vi "MFCConfigurationGlobal.vi"(6 "Index":i32, 7 "Action":T5=enum."Get", 11 "Set Value":T1) -> (3 "Value Out":T1)   [LabVIEW 2012]
uses:
  MFCConfigurationGlobalAction.ctl
  MFCConfiguration.ctl
  libs/Sierra-M100/Public/Controls/ValveState.ctl
  libs/Sierra-M100/Public/Controls/Gas.ctl
  libs/Sierra-M100/Public/Controls/Units.ctl
  libs/Sierra-M100/Sierra-M100.lvlib
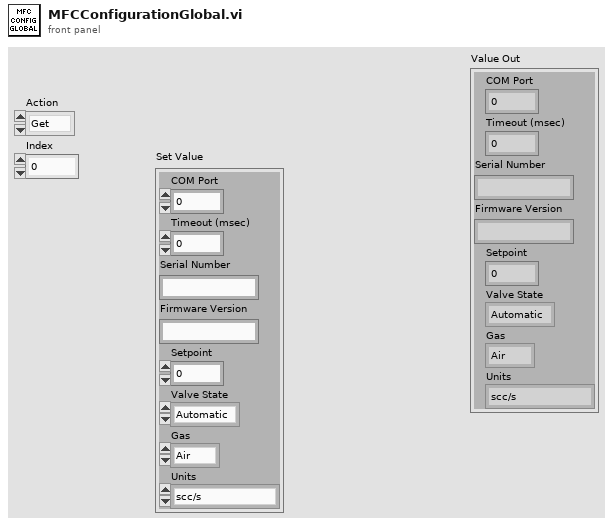
[diagram p1: front panel]
types:
  T1 = typedef "MFCConfiguration.ctl" = cluster{"COM Port":u32, "Timeout (msec)":u32, "Setpoint":dbl, "Valve State":T2, "Gas":T3, "Units":T4, "Serial Number":string, "Firmware Version":string}
  T2 = typedef "Sierra-M100.lvlib/ValveState.ctl" = enum16{"Automatic", "Closed", "Purge"}
  T3 = typedef "Sierra-M100.lvlib/Gas.ctl" = enum16{"Air", "Argon", "CO2", "CO", "Helium", "Hydrogen", "Methane", "Nitrogen", "Nitrous Oxide", "Oxygen"}
  T4 = typedef "Sierra-M100.lvlib/Units.ctl" = enum16{"scc/s", "scc/m", "scc/H", "Ncc/s", "Ncc/m", "Ncc/H", "SCF/s", "SCF/m", "SCF/H", "NM3/s", "NM3/m", "NM3/H", "SM3/s", "SM3/m", "SM3/H", "sl/s", "sl/m", "sl/H", "NL/s", "NL/m", "Nl/H", "g/s", "g/m", "g/H", "kg/s", "kg/m", "kg/H", "lb/s", "lb/m", "lb/H"}
  T5 = typedef "MFCConfigurationGlobalAction.ctl" = enum16{"Init", "Get", "Set", "Add", "Remove", "Reset"}
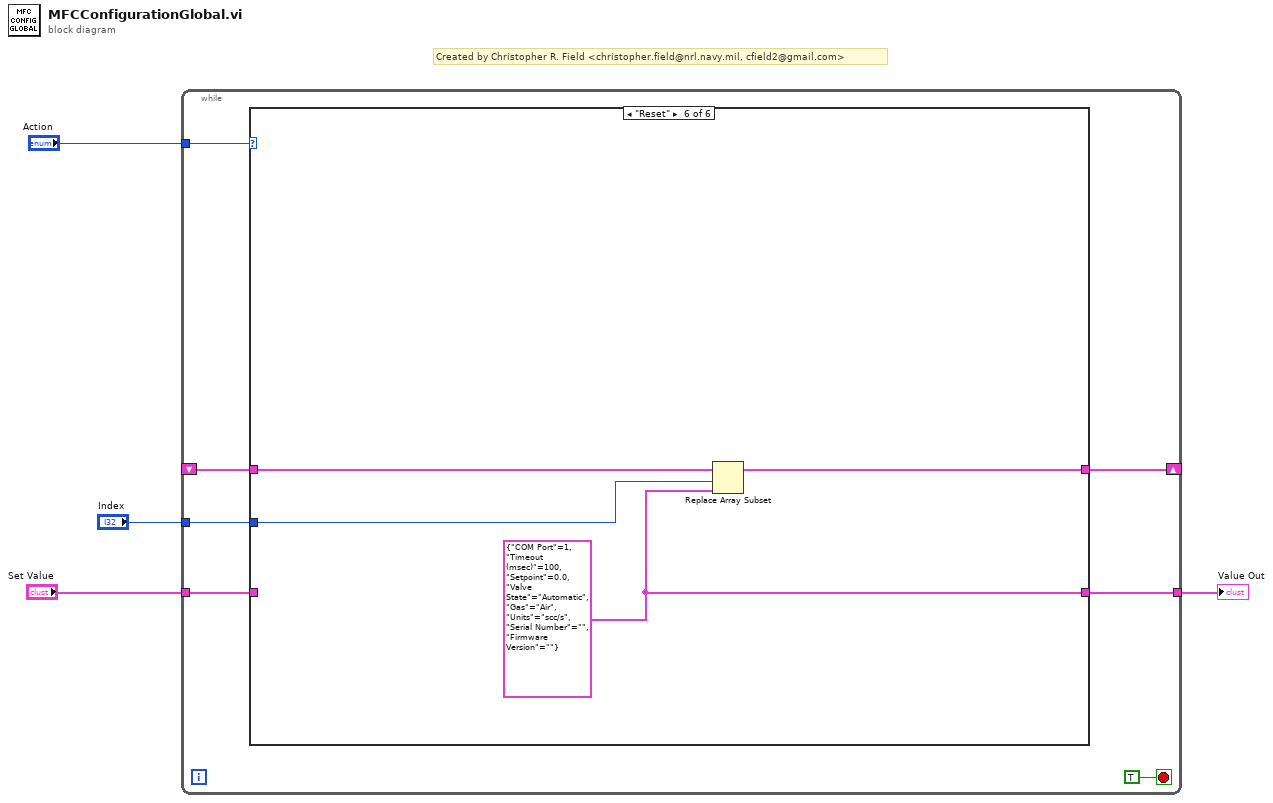
[diagram p0: block diagram]
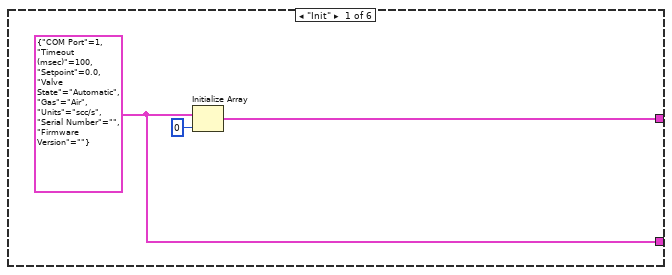
[diagram p2: hidden frame]
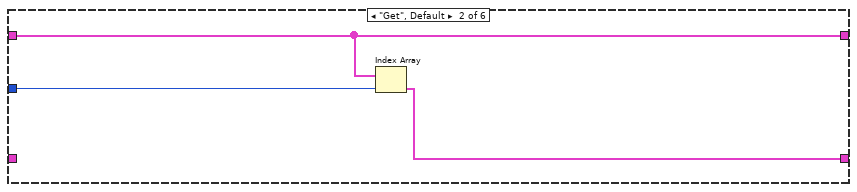
[diagram p3: hidden frame]
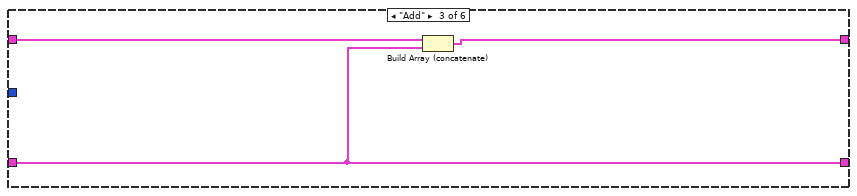
[diagram p4: hidden frame]
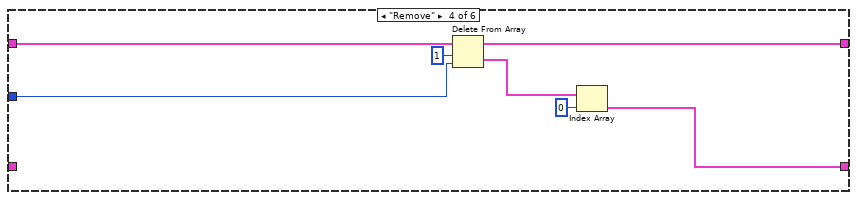
[diagram p5: hidden frame]
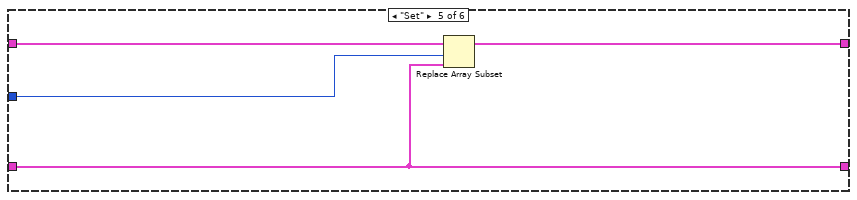
[diagram p6: hidden frame]
diagram:
  # "Created by Christopher R. Field <christopher.field@nrl.navy.mil, cfield2@gmail.com>"
  n1 = while {
    tunnel: "Action" -> [w10]
    tunnel: "Set Value" -> [w9]
    shift-right: [w7] -> _
    shift-left: _ -> [w8]
    tunnel: [w6] -> w2
    tunnel: "Index" -> [w5]
    stop <- TRUE stop-if-true
    n2 = case shown="\"Reset\"" w10 {
      tunnel: w9 -> [_ _ w19 _ w28 _]
      tunnel: w8 -> [_ w17 w20 w27 w31 w35]
      tunnel: [w13 w17 w18 w26 w30 w34] -> w7
      tunnel: [w12 w15 w19 w21 w28 w32] -> w6
      tunnel: w5 -> [_ w16 _ w23 w29 w33]
      frame "Init" {
        w12 = T1 {"COM Port"=1, "Timeout (msec)"=100, "Setpoint"=0.0, "Valve State"=enum."Automatic", "Gas"=enum."Air", "Units"=enum."scc/s", "Serial Number"="", "Firmware Version"=""} ("Set Value")
        n3 = Initialize Array(w12, 0 ("dimension size")) -> (w13:T1[])
      }
      frame "Get", Default {
        n4 = Index Array(array=w17, index=w16) -> (element=w15:T1)
      }
      frame "Add" {
        n5 = Build Array (concatenate)(w20, w19) -> (w18:T1[])
      }
      frame "Remove" {
        n6 = Delete From Array(array=w27, length=1, index=w23) -> (deleted portion=w25:T1[], array with subset deleted=w26:T1[])
        n7 = Index Array(array=w25, index=0) -> (element=w21:T1)
      }
      frame "Set" {
        n8 = Replace Array Subset(array=w31, new element=w28, index=w29) -> (w30:T1[])
      }
      frame "Reset" {
        w32 = T1 {"COM Port"=1, "Timeout (msec)"=100, "Setpoint"=0.0, "Valve State"=enum."Automatic", "Gas"=enum."Air", "Units"=enum."scc/s", "Serial Number"="", "Firmware Version"=""} ("Set Value")
        n9 = Replace Array Subset(array=w35, new element=w32, index=w33) -> (w34:T1[])
      }
    }
  }
  "Value Out" <- w2
